vi "Rework_Calculate.vi"(9 "Rework站号":string, 10 "当前站号":string) -> (1 "Data":string[](array[string]), 2 "Rework_List":string[](array[string]), 3 "跨站":bool)   [LabVIEW 2018]
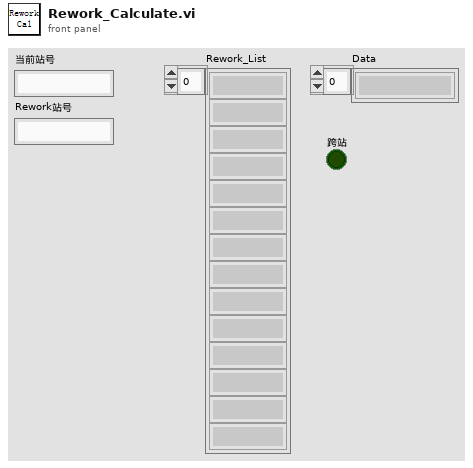
[diagram p1: front panel]
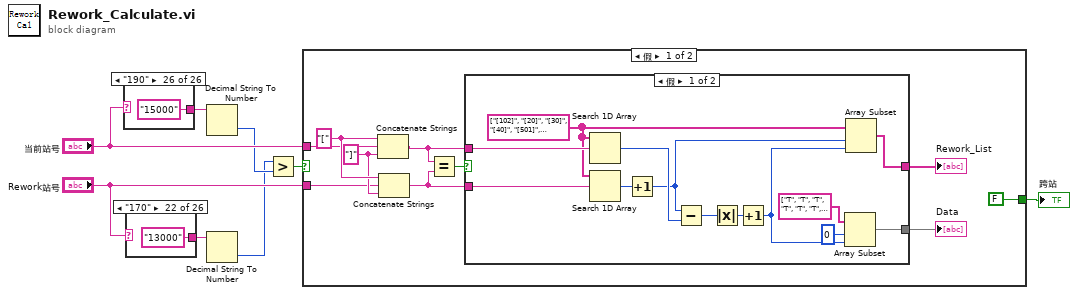
[diagram p0: block diagram]
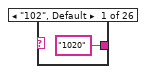
[diagram p2: hidden frame]
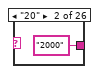
[diagram p3: hidden frame]
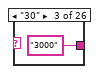
[diagram p4: hidden frame]
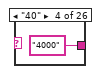
[diagram p5: hidden frame]
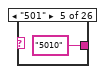
[diagram p6: hidden frame]
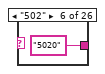
[diagram p7: hidden frame]
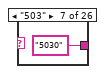
[diagram p8: hidden frame]
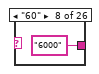
[diagram p9: hidden frame]
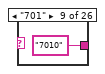
[diagram p10: hidden frame]
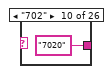
[diagram p11: hidden frame]
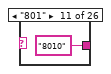
[diagram p12: hidden frame]
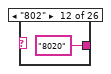
[diagram p13: hidden frame]
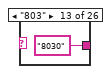
[diagram p14: hidden frame]
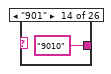
[diagram p15: hidden frame]
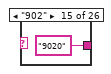
[diagram p16: hidden frame]
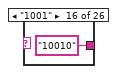
[diagram p17: hidden frame]
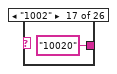
[diagram p18: hidden frame]
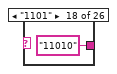
[diagram p19: hidden frame]
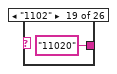
[diagram p20: hidden frame]
diagram:
  n1 = case shown="\"190\"" "当前站号" {
    tunnel: ["1020" "2000" "3000" "4000" "5010" "5020" "5030" "6000" "7010" "7020" "8010" "8020" "8030" "9010" "9020" "10010" "10020" "11010" "11020" "12000" "13000" "13000" "14000" "14000" "15000" "15000"] -> w5
    frame "102", Default {
    }
    frame "20" {
    }
    frame "30" {
    }
    frame "40" {
    }
    frame "501" {
    }
    frame "502" {
    }
    frame "503" {
    }
    frame "60" {
    }
    frame "701" {
    }
    frame "702" {
    }
    frame "801" {
    }
    frame "802" {
    }
    frame "803" {
    }
    frame "901" {
    }
    frame "902" {
    }
    frame "1001" {
    }
    frame "1002" {
    }
    frame "1101" {
    }
    frame "1102" {
    }
    frame "120" {
    }
    frame "130" {
    }
    frame "170" {
    }
    frame "140" {
    }
    frame "180" {
    }
    frame "150" {
    }
    frame "190" {
    }
  }
  n2 = case shown="\"170\"" "Rework站号" {
    tunnel: ["1020" "2000" "3000" "4000" "5010" "5020" "5030" "6000" "7010" "7020" "8010" "8020" "8030" "9010" "9020" "10010" "10020" "11010" "11020" "12000" "13000" "13000" "14000" "14000" "15000" "15000"] -> w3
    frame "102", Default {
    }
    frame "20" {
    }
    frame "30" {
    }
    frame "40" {
    }
    frame "501" {
    }
    frame "502" {
    }
    frame "503" {
    }
    frame "60" {
    }
    frame "701" {
    }
    frame "702" {
    }
    frame "801" {
    }
    frame "802" {
    }
    frame "803" {
    }
    frame "901" {
    }
    frame "902" {
    }
    frame "1001" {
    }
    frame "1002" {
    }
    frame "1101" {
    }
    frame "1102" {
    }
    frame "120" {
    }
    frame "130" {
    }
    frame "170" {
    }
    frame "140" {
    }
    frame "180" {
    }
    frame "150" {
    }
    frame "190" {
    }
  }
  n3 = Decimal String To Number(string=w5) -> (number=w4:i32)  [unwired: 2 in, 1 out]
  n4 = Decimal String To Number(string=w3) -> (number=w2:i32)  [unwired: 2 in, 1 out]
  n5 = Greater?(x=w2, y=w4) -> (0:w1:bool)
  n6 = case shown="假" w1 {
    tunnel: "当前站号" -> [w63 _]
    tunnel: "Rework站号" -> [w62 _]
    tunnel: [FALSE TRUE] -> w8
    frame False {
      w64 = "]" ("字符串")
      w65 = "[" ("字符串")
      n7 = Concatenate Strings(w65, w63, w64) -> (w67:string)
      n8 = Concatenate Strings(w65, w62, w64) -> (w66:string)
      n9 = Equal?(x=w67, y=w66) -> (x = y?=w70:bool)
      n10 = case shown="假" w70 {
        tunnel: w66 -> [w82 w88]
        tunnel: [w79 w85] -> w69
        tunnel: [w72 string[] ["T"]] -> w68
        tunnel: w67 -> [w83 _]
        frame False {
          w71 = string[] ["[102]", "[20]", "[30]", "[40]", "[501]", "[502]", "[503]", "[60]", "[701]", "[702]", "[801]", "[802]", "[803]", "[901]", "[902]", "[1001]", "[1002]", "[1101]", "[1102]", "[120]", "[130]", "[170]", "[140]", "[180]", "[150]", "[190]"]
          n11 = Search 1D Array(1D array=w71, element=w83) -> (index of element=w81:i32)  [unwired: 1 in]
          n12 = Search 1D Array(1D array=w71, element=w82) -> (index of element=w75:i32)  [unwired: 1 in]
          n13 = Increment(x=w75) -> (x+1=w74:i32)
          n14 = Subtract(x=w74, y=w81) -> (x-y=w80:i32)
          n15 = Absolute Value(x=w80) -> (abs(x)=w77:i32)
          n16 = Increment(x=w77) -> (x+1=w76:i32)
          n17 = Array Subset(array=string[] ["T", "T", "T", "T", "T", "T", "T", "T", "T", "T", "T", "T", "T", "T", "T", "T", "T", "T", "T", "T", "T", "T", "T", "T", "T", "T"], index=0 ("索引"), length=w76) -> (w72:string[])
          n18 = Array Subset(array=w71, index=w74, length=w76) -> (w79:string[])
        }
        frame True {
          n19 = Insert Into Array(array=string[] [] ("数组"), index=0 ("索引"), new element=w88) -> (w85:string[])
        }
      }
      "Rework_List" <- w69
      "Data" <- w68
    }
    frame True {
    }
  }
  "跨站" <- w8
